vi "Recurse Through Project Items.vi"(6 "FPGA":string, 7 "FPGA Resource":string, 8 "error in (no error)":errorcluster, 9 "IO in":variant, 10 "Modules in":variant, 11 "ProjectItem in":refnum<vi>) -> (0 "error out":errorcluster, 1 "IO out":variant, 2 "Modules out":variant)   [LabVIEW 2015, in "Project.lvclass"]
uses:
  Project.lvclass
  Elemental IO Properties.ctl
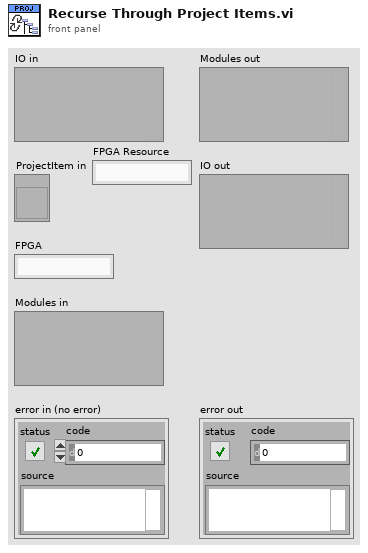
[diagram p1: front panel]
types:
  T1 = typedef "Project.lvclass/Elemental IO Properties.ctl" = cluster{"FPGA Name":string, "Mod":string, "IO Resource":string, "IO Name":string, "FPGA Resource":string}
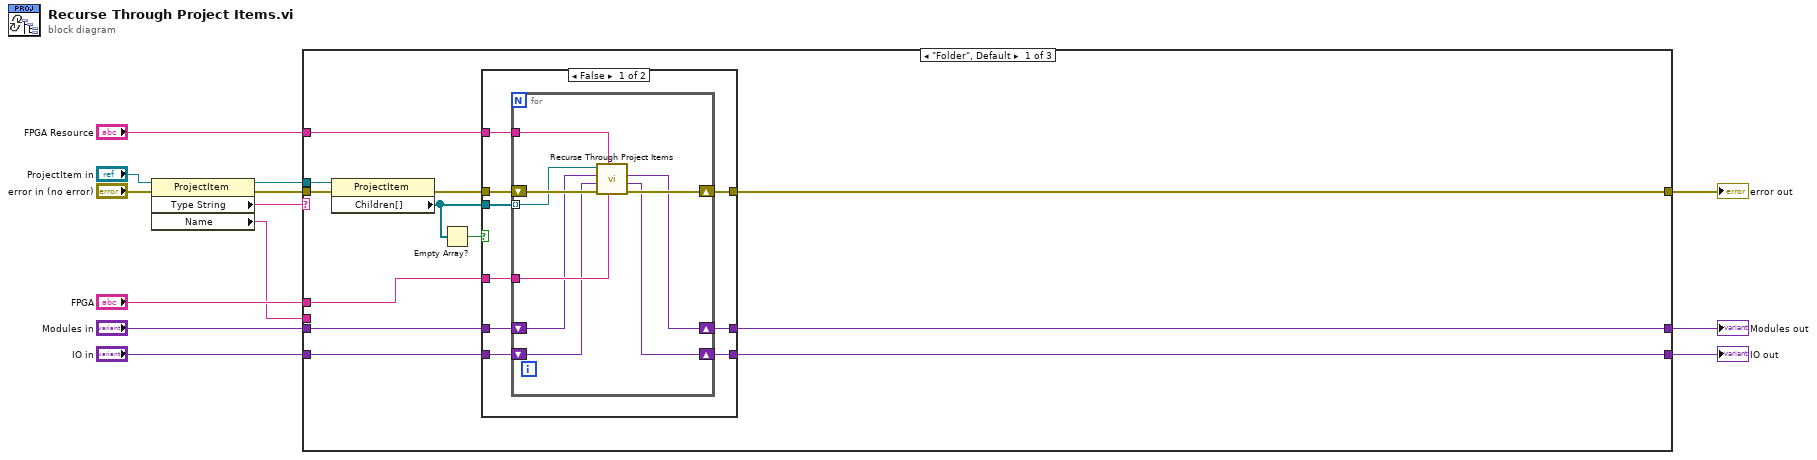
[diagram p0: block diagram]
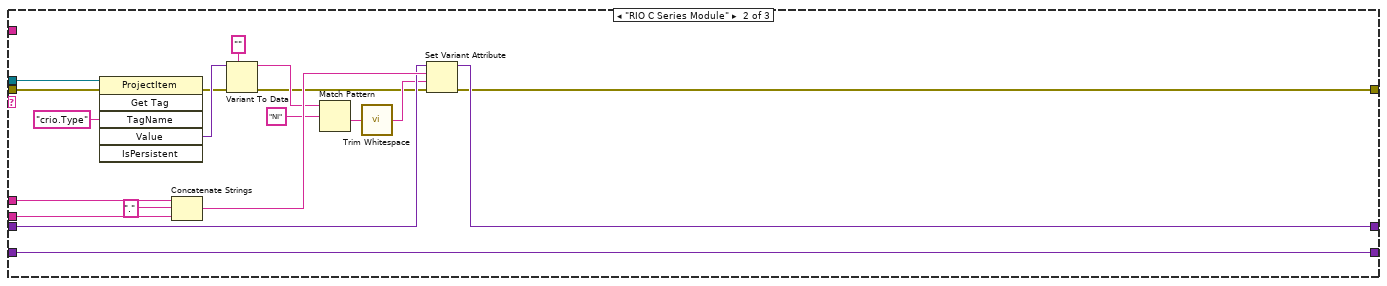
[diagram p3: hidden frame]
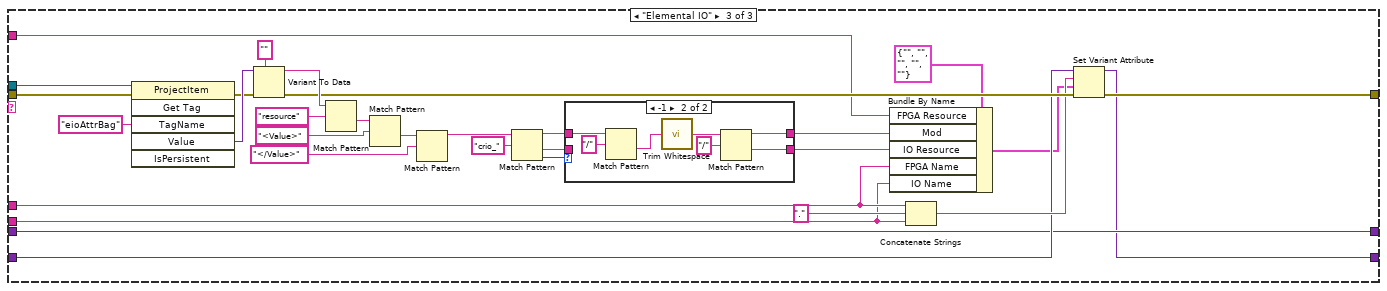
[diagram p4: hidden frame]
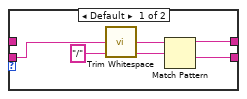
[diagram p5: hidden frame]
diagram:
  n1 = property class="ProjectItem"(reference="ProjectItem in", error in="error in (no error)") -> (reference out=w5:refnum<vi>, error out=w6:errorcluster, "Type String"=w4:string, "Name"=w8:string)
  n2 = case shown="\"Folder\", Default" w4 {
    tunnel: w5 -> [w25 w65 w96]
    tunnel: w6 -> [w24 w63 w95]
    tunnel: [w20 w48 w83] -> w7
    tunnel: w8 -> [_ w57 w72]
    tunnel: "FPGA" -> [w19 w59 w74]
    tunnel: "Modules in" -> [w18 w55 w80]
    tunnel: [w15 w54 w80] -> w11
    tunnel: "IO in" -> [w17 w47 w81]
    tunnel: [w16 w47 w79] -> w13
    tunnel: "FPGA Resource" -> [w14 _ w66]
    frame "Folder", Default {
      n3 = property class="ProjectItem"(reference=w25, error in=w24) -> (error out=w22:errorcluster, "Children[]"=w21:refnum<vi>[])  [unwired: 1 out]
      n4 = Empty Array?(array=w21) -> (empty?=w23:bool)
      n5 = case shown="False" w23 {
        tunnel: w22 -> [w34 w46]
        tunnel: w21 -> [w33 _]
        tunnel: [w32 w46] -> w20
        tunnel: w19 -> [w31 _]
        tunnel: w18 -> [w30 w44]
        tunnel: w17 -> [w29 w45]
        tunnel: [w28 w45] -> w16
        tunnel: [w27 w44] -> w15
        tunnel: w14 -> [w26 _]
        frame False {
          n6 = for {
            tunnel: w33 -> [w42] mode=indexing
            shift-right: [w40] -> w32
            shift-left: w34 -> [w43]
            tunnel: w31 -> [w41]
            shift-right: [w36] -> w27
            shift-left: w30 -> [w39]
            shift-right: [w37] -> w28
            shift-left: w29 -> [w38]
            tunnel: w26 -> [w35]
            n7 = call "Recurse Through Project Items.vi"("FPGA"=w41, "FPGA Resource"=w35, "error in (no error)"=w43, "IO in"=w38, "Modules in"=w39, "ProjectItem in"=w42) -> ("error out"=w40:errorcluster, "IO out"=w37:variant, "Modules out"=w36:variant)  [unwired: 3 in]
          }
        }
        frame True {
        }
      }
    }
    frame "RIO C Series Module" {
      n8 = invoke class="ProjectItem" method="Get Tag"(reference=w65, error in=w63, "TagName"="crio.Type" ("Tag Name")) -> (error out=w61:errorcluster, "Value"=w62:variant)  [unwired: 3 in, 4 out]
      n9 = Concatenate Strings(w59, "." ("string"), w57) -> (w56:string)
      n10 = Variant To Data(error in=w61, type="", Variant=w62) -> (data=w53:string, error out=w49:errorcluster)
      n11 = Match Pattern(string=w53, regular expression="NI") -> (after substring=w52:string)  [unwired: 1 in, 3 out]
      n12 = call <vilib>:"Trim Whitespace.vi"("string"=w52) -> ("trimmed string"=w50:string)  [unwired: 1 in]
      n13 = Set Variant Attribute(Variant=w55, name=w56, value=w50, error in=w49) -> (Variant out=w54:variant, error out=w48:errorcluster)  [unwired: 1 out]
    }
    frame "Elemental IO" {
      n14 = invoke class="ProjectItem" method="Get Tag"(reference=w96, error in=w95, "TagName"="eioAttrBag" ("Tag Name")) -> (error out=w90:errorcluster, "Value"=w93:variant)  [unwired: 3 in, 4 out]
      n15 = Variant To Data(error in=w90, type="" ("Tag Name"), Variant=w93) -> (data=w91:string, error out=w84:errorcluster)
      n16 = Match Pattern(string=w91, regular expression="resource") -> (after substring=w88:string)  [unwired: 1 in, 3 out]
      n17 = Match Pattern(string=w88, regular expression="<Value>") -> (after substring=w86:string)  [unwired: 1 in, 3 out]
      n18 = Match Pattern(string=w86, regular expression="</Value>") -> (before substring=w71:string)  [unwired: 1 in, 3 out]
      n19 = Match Pattern(string=w71, regular expression="crio_") -> (before substring=w67:string, after substring=w68:string, offset past match=w69:i32)  [unwired: 1 in, 1 out]
      n20 = case shown="-1" w69 {
        tunnel: [w99 w106] -> w76
        tunnel: [w98 w105] -> w75
        tunnel: w68 -> [w97 _]
        tunnel: w67 -> [_ w102]
        frame Default {
          n21 = call <vilib>:"Trim Whitespace.vi"("string"=w97) -> ("trimmed string"=w101:string)  [unwired: 1 in]
          n22 = Match Pattern(string=w101, regular expression="/") -> (before substring=w99:string, after substring=w98:string)  [unwired: 1 in, 2 out]
        }
        frame -1 {
          n23 = Match Pattern(string=w102, regular expression="/") -> (after substring=w103:string)  [unwired: 1 in, 3 out]
          n24 = call <vilib>:"Trim Whitespace.vi"("string"=w103) -> ("trimmed string"=w108:string)  [unwired: 1 in]
          n25 = Match Pattern(string=w108, regular expression="/") -> (before substring=w106:string, after substring=w105:string)  [unwired: 1 in, 2 out]
        }
      }
      n26 = Bundle By Name(cluster=T1 {"FPGA Name"="", "Mod"="", "IO Resource"="", "IO Name"="", "FPGA Resource"=""}, "FPGA Resource"=w66, "Mod"=w76, "IO Resource"=w75, "FPGA Name"=w74, "IO Name"=w72) -> (w73:T1)
      n27 = Concatenate Strings(w74, "." ("string"), w72) -> (w82:string)
      n28 = Set Variant Attribute(Variant=w81, name=w82, value=w73, error in=w84) -> (Variant out=w79:variant, error out=w83:errorcluster)  [unwired: 1 out]
    }
  }
  "IO out" <- w13
  "Modules out" <- w11
  "error out" <- w7
